vi "(10) Move XY (Stop and Scan) - Automatic Loop.vi"() -> ()   [LabVIEW 2020]
uses:
  <instrlib>/Arcus Ethernet Driver 1.0.0/ArcusEthernetComm/classes/Controller/_Controller.lvclass
panel:
  in  "Y Diirection":bool
  in  "Y Desired Increment (mm)":dbl
  in  "Initial Direction":bool
  in  "X Desired Distance (mm)":dbl
  in  "error in (no error)":errorcluster
  in  "Scan":bool
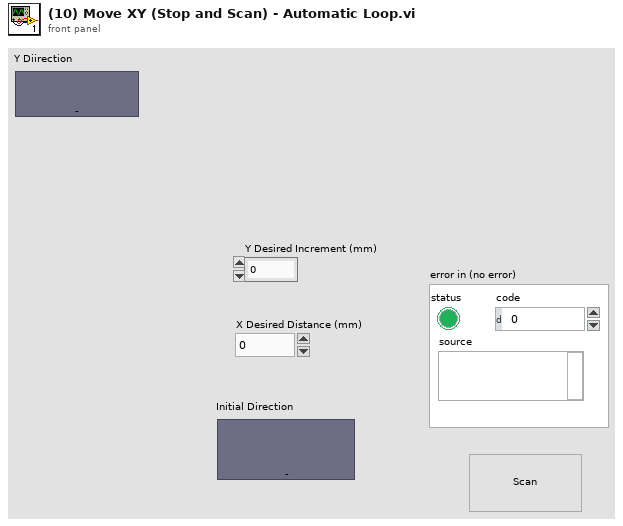
[diagram p1: front panel]
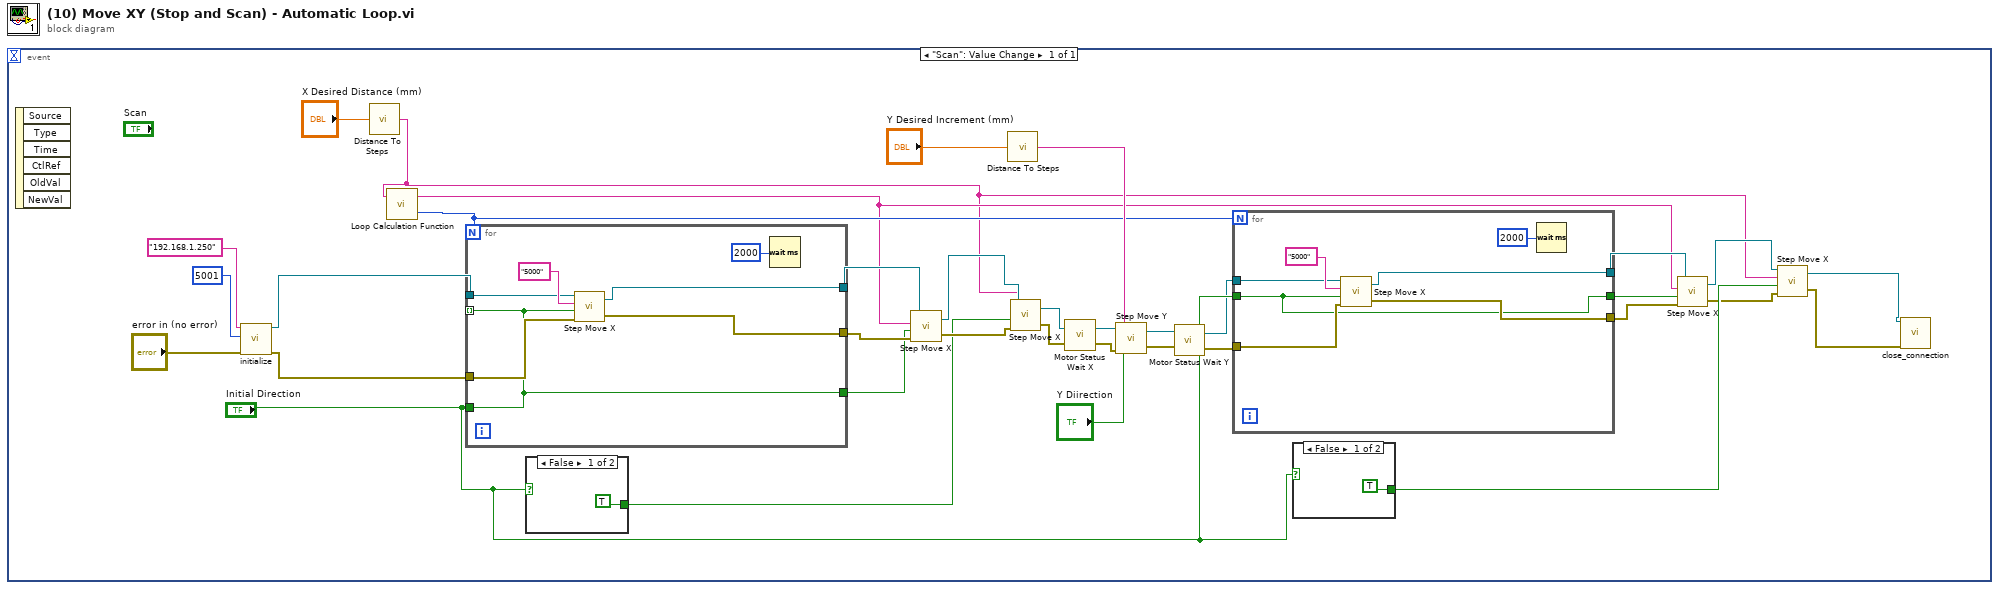
[diagram p0: block diagram]
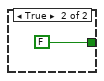
[diagram p2: hidden frame]
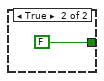
[diagram p3: hidden frame]
diagram:
  n1 = event shown="[0] \"Scan\": Value Change" {
    selector: _ -> [_]
    dyn-events: _ -> [_]
    timeout: _ -> [_]
    event "Scan": Value Change {
      n2 = event-data() -> ()  [unwired: 1 in, 6 out]
      n3 = call <instrlib>:"initialize.vi"("ip_address (in)"="192.168.1.250", "dev_port(def=5001)"=u16 5001, "error in (no error)"="error in (no error)") -> ("reference (out)"=w30:refnum<class "_Controller.lvclass">, "error out"=w31:errorcluster)  [unwired: 15 in]
      n4 = call "Distance To Steps.vi"("Desired Distance (mm)"="X Desired Distance (mm)") -> ("Number of Steps"=w14:string)
      n5 = call "Loop Calculation Function.vi"("Number of Steps"=w14) -> ("No. of Loops (-1)"=w16:i32, "Remainder"=w15:string)  [unwired: 1 in]
      n6 = for {
        N: w16 -> [_]
        tunnel: w31 -> [w51]
        tunnel: [w49] -> w29
        tunnel: [w47] -> _ mode=indexing
        tunnel: "Initial Direction" -> [w47]
        tunnel: w30 -> [w50]
        tunnel: [w48] -> w28
        tunnel: [w47] -> w27
        n7 = call "Step Move X.vi"("error in (no error)"=w51, "Direction"=w47, "x steps"="5000" ("X Steps"), "reference (in)"=w50) -> ("error out"=w48:errorcluster, "reference (out)"=w49:refnum<class "_Controller.lvclass">)
        n8 = Wait (ms)(milliseconds to wait=u32 2000) -> ()  [unwired: 1 out]
      }
      n9 = case shown="False" "Initial Direction" {
        tunnel: [TRUE FALSE] -> w24
        frame False {
        }
        frame True {
        }
      }
      n10 = call "Step Move X.vi"("error in (no error)"=w28, "Direction"=w27, "x steps"=w15, "reference (in)"=w29) -> ("error out"=w25:errorcluster, "reference (out)"=w26:refnum<class "_Controller.lvclass">)
      n11 = call "Distance To Steps.vi"("Desired Distance (mm)"="Y Desired Increment (mm)") -> ("Number of Steps"=w23:string)
      n12 = call "Step Move X.vi"("error in (no error)"=w25, "Direction"=w24, "x steps"=w14, "reference (in)"=w26) -> ("error out"=w4:errorcluster, "reference (out)"=w5:refnum<class "_Controller.lvclass">)
      n13 = call "Motor Status Wait X.vi"("error in"=w4, "reference (in)"=w5) -> ("error out"=w6:errorcluster, "reference (out)"=w7:refnum<class "_Controller.lvclass">)
      n14 = call "Step Move Y.vi"("error in (no error)"=w6, "Direction"="Y Diirection", "Y Steps"=w23, "reference (in)"=w7) -> ("error out"=w9:errorcluster, "reference (out)"=w10:refnum<class "_Controller.lvclass">)
      n15 = call "Motor Status Wait Y.vi"("error in"=w9, "reference (in)"=w10) -> ("error out 2"=w8:errorcluster, "reference (out) 2"=w11:refnum<class "_Controller.lvclass">)
      n16 = for {
        N: w16 -> [_]
        tunnel: [w42] -> w17
        tunnel: [w41] -> w18
        tunnel: w11 -> [w40]
        tunnel: w8 -> [w39]
        tunnel: "Initial Direction" -> [w38]
        tunnel: [w38] -> w13
        n17 = call "Step Move X.vi"("error in (no error)"=w39, "Direction"=w38, "x steps"="5000" ("X Steps"), "reference (in)"=w40) -> ("error out"=w41:errorcluster, "reference (out)"=w42:refnum<class "_Controller.lvclass">)
        n18 = Wait (ms)(milliseconds to wait=u32 2000) -> ()  [unwired: 1 out]
      }
      n19 = case shown="False" "Initial Direction" {
        tunnel: [TRUE FALSE] -> w21
        frame False {
        }
        frame True {
        }
      }
      n20 = call "Step Move X.vi"("error in (no error)"=w18, "Direction"=w13, "x steps"=w15, "reference (in)"=w17) -> ("error out"=w20:errorcluster, "reference (out)"=w19:refnum<class "_Controller.lvclass">)
      n21 = call "Step Move X.vi"("error in (no error)"=w20, "Direction"=w21, "x steps"=w14, "reference (in)"=w19) -> ("error out"=w1:errorcluster, "reference (out)"=w2:refnum<class "_Controller.lvclass">)
      n22 = call <instrlib>:"close_connection.vi"("reference (in)"=w2, "error in (no error)"=w1) -> ()  [unwired: 16 in, 2 out]
    }
  }
